vi "HEALTH_LABVIEW_V3.vi"() -> ()   [LabVIEW 2026]
panel:
  out "Waveform Chart":dbl(graph)
  in  "HTR PROP GAIN":dbl=3.0
  in  "PUMP SPEED CONTROL VOLTAGE":dbl(knob) scale=0.0..5.0
  in  "TARGET COOLANT FLOW RATE (LPM)":dbl
  in  "PUMP ON/OFF":bool
  out "HEATER TEMPERATURE (C)":dbl(graph)
  out "HEATER POWER OUTPUT":dbl(knob) scale=0.0..100.0
  in  "TARGET HEATER TEMP (C)":dbl
  in  "HEATER ON/OFF":bool
  out "HEATER TEMP (C)":dbl(knob) scale=20.0..90.0
  out "HEATER TEMP (C)":dbl format="%.2f"
  in  "stop":bool
  out "Error String":string
  out "error out":errorcluster
  out "ConnectionType Out":i32
  out "DeviceType Out":i32
  in  "Identifier":string="LJM_idANY"
  in  "ConnectionType":string="LJM_ctANY"
  in  "DeviceType":string="LJM_dtANY"
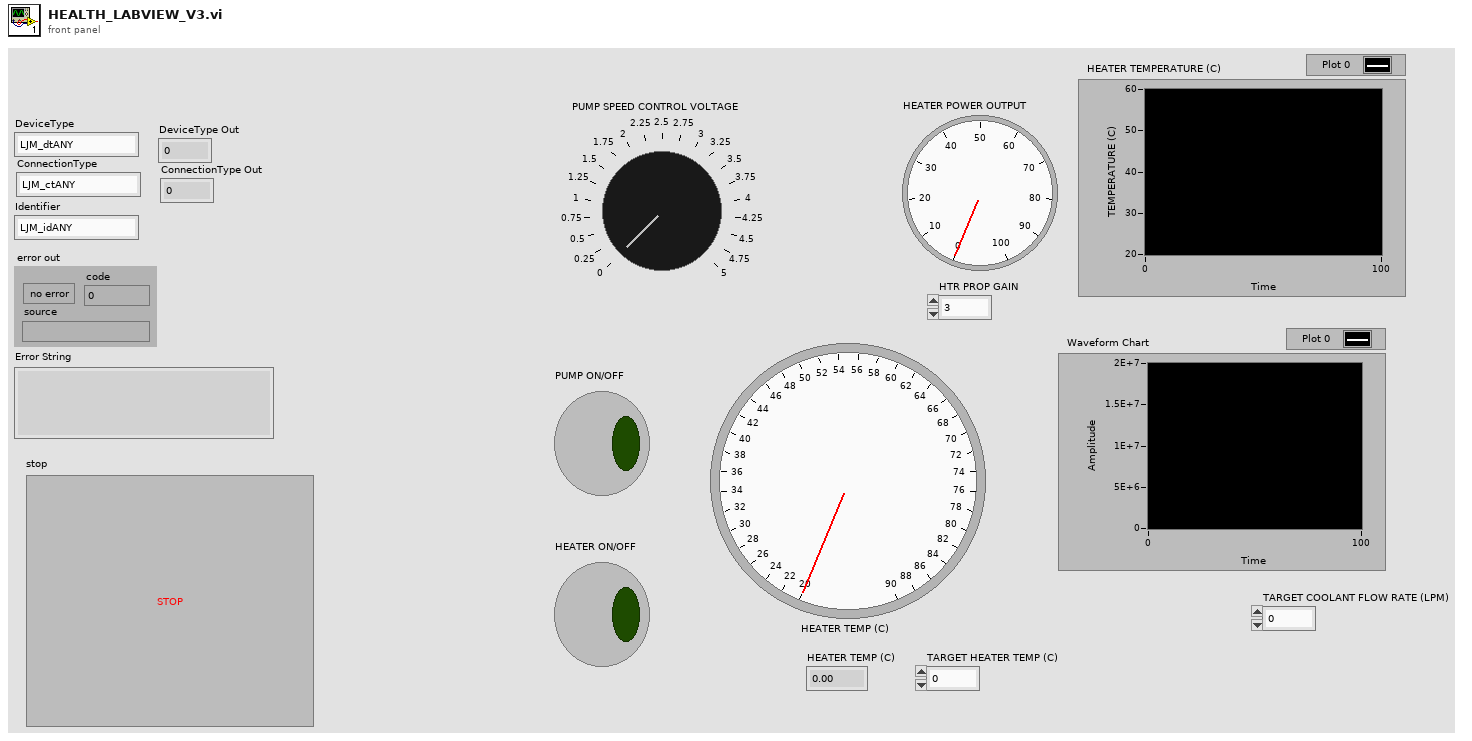
[diagram p1: front panel]
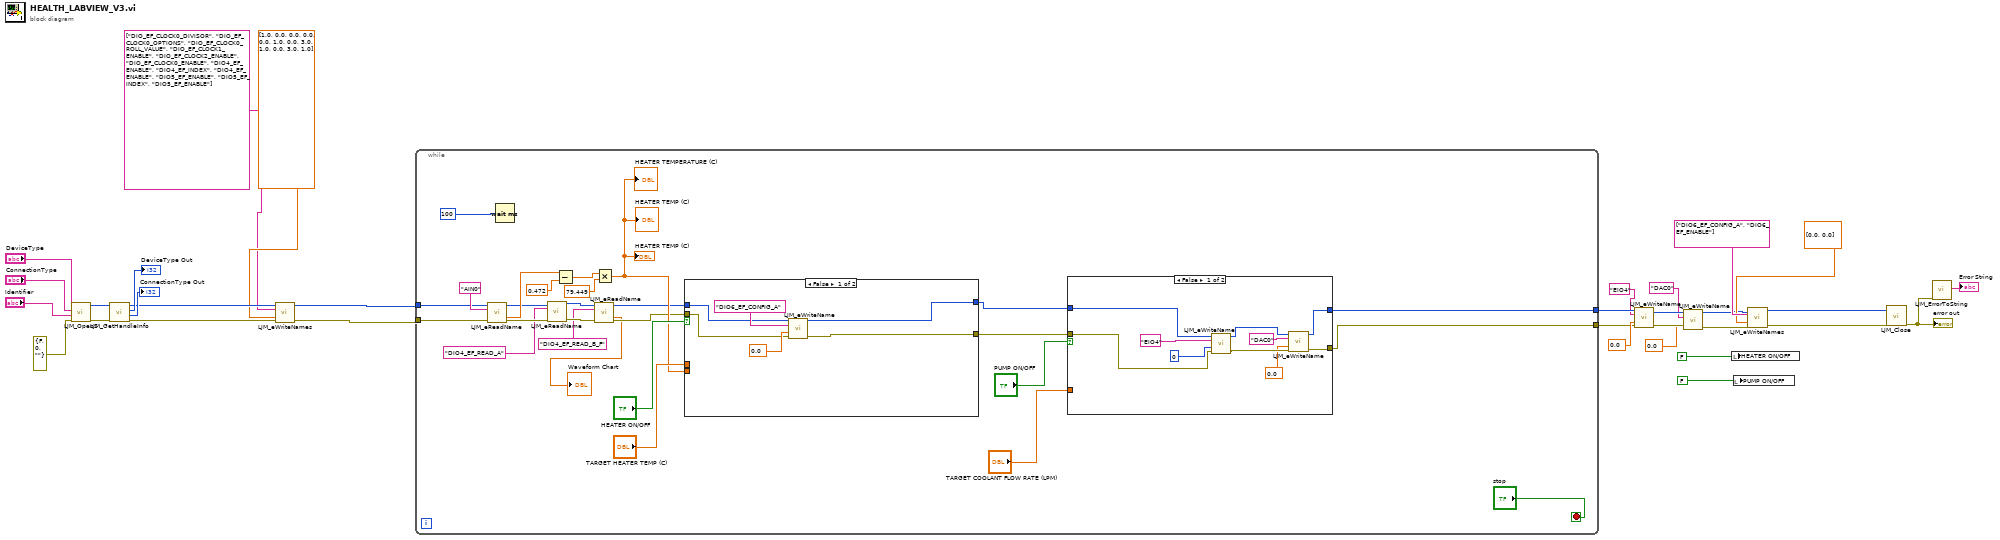
[diagram p0: block diagram]
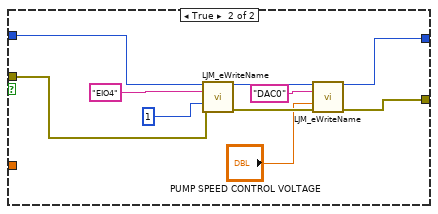
[diagram p2: hidden frame]
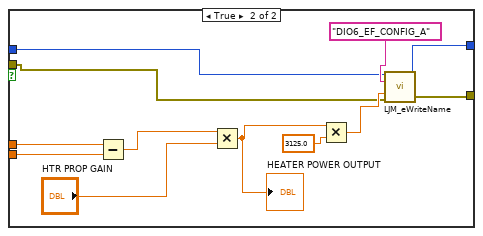
[diagram p3: hidden frame]
diagram:
  n1 = call "LJM_OpenS.vi"("error in"=errorcluster {"status"=FALSE, "code"=0, "source"=""} ("error in (no error)"), "Identifier"="Identifier", "ConnectionType"="ConnectionType", "DeviceType"="DeviceType") -> ("error out"=w31:errorcluster, "Handle"=w30:i32)  [unwired: 6 in]
  n2 = call "LJM_GetHandleInfo.vi"("error in"=w31, "Handle In"=w30) -> ("error out"=w21:errorcluster, "ConnectionType"=→"ConnectionType Out":i32, "DeviceType"=→"DeviceType Out":i32, "Handle Out"=w22:i32)  [unwired: 2 in, 4 out]
  n3 = call "LJM_eWriteNames.vi"("Handle In"=w22, "aNames"=string[] ["DIO_EF_CLOCK0_DIVISOR", "DIO_EF_CLOCK0_OPTIONS", "DIO_EF_CLOCK0_ROLL_VALUE", "DIO_EF_CLOCK1_ENABLE", "DIO_EF_CLOCK2_ENABLE", "DIO_EF_CLOCK0_ENABLE", "DIO4_EF_ENABLE", "DIO4_EF_INDEX", "DIO4_EF_ENABLE", "DIO5_EF_ENABLE", "DIO5_EF_INDEX", "DIO5_EF_ENABLE"], "aValuesIn"=dbl[] [1.0, 0.0, 0.0, 0.0, 0.0, 1.0, 0.0, 3.0, 1.0, 0.0, 3.0, 1.0], "error in"=w21) -> ("Handle Out"=w2:i32, "error out"=w1:errorcluster)  [unwired: 9 in, 1 out]
  n4 = while {
    tunnel: [w45] -> w9
    tunnel: w2 -> [w44]
    tunnel: w1 -> [w43]
    tunnel: [w42] -> w3
    stop <- "stop" stop-if-true
    n5 = call "LJM_eReadName.vi"("Handle In"=w44, "Name"="AIN0", "error in"=w43) -> ("Handle Out"=w41:i32, "Value"=w55:dbl, "error out"=w40:errorcluster)  [unwired: 10 in]
    n6 = Wait (ms)(milliseconds to wait=u32 100) -> ()  [unwired: 1 out]
    n7 = call "LJM_eReadName.vi"("Handle In"=w41, "Name"="DIO4_EF_READ_A", "error in"=w40) -> ("Handle Out"=w39:i32, "error out"=w38:errorcluster)  [unwired: 10 in, 1 out]
    n8 = Subtract(x=w55, y=0.472 ("Address 2")) -> (x-y=w58:dbl)
    n9 = call "LJM_eReadName.vi"("Handle In"=w39, "Name"="DIO4_EF_READ_B_F", "error in"=w38) -> ("Handle Out"=w37:i32, "Value"=→"Waveform Chart":dbl, "error out"=w36:errorcluster)  [unwired: 10 in]
    n10 = Multiply(x=w58, y=79.449 ("Address 2")) -> (x*y=w50:dbl)
    "HEATER TEMP (C)" <- w50
    "HEATER TEMP (C)" <- w50
    "HEATER TEMPERATURE (C)" <- w50
    n11 = case shown="False" "HEATER ON/OFF" {
      tunnel: [w84 w97] -> w46
      tunnel: [w85 w96] -> w47
      tunnel: "TARGET HEATER TEMP (C)" -> [_ w92]
      tunnel: w50 -> [_ w91]
      tunnel: w37 -> [w81 w87]
      tunnel: w36 -> [w80 w86]
      frame False {
        n12 = call "LJM_eWriteName.vi"("Handle In"=w81, "Name"="DIO6_EF_CONFIG_A", "Value"=0.0, "error in"=w80) -> ("Handle Out"=w85:i32, "error out"=w84:errorcluster)  [unwired: 10 in]
      }
      frame True {
        n13 = Subtract(x=w92, y=w91) -> (x-y=w89:dbl)
        n14 = Multiply(x=w89, y="HTR PROP GAIN") -> (x*y=w88:dbl)
        "HEATER POWER OUTPUT" <- w88
        n15 = Multiply(x=w88, y=3125.0) -> (x*y=w94:dbl)
        n16 = call "LJM_eWriteName.vi"("Handle In"=w87, "Name"="DIO6_EF_CONFIG_A", "Value"=w94, "error in"=w86) -> ("Handle Out"=w96:i32, "error out"=w97:errorcluster)  [unwired: 10 in]
      }
    }
    n17 = case shown="False" "PUMP ON/OFF" {
      tunnel: "TARGET COOLANT FLOW RATE (LPM)" -> [_ _]
      tunnel: w47 -> [w67 w77]
      tunnel: w46 -> [w66 w76]
      tunnel: [w62 w71] -> w42
      tunnel: [w61 w72] -> w45
      frame False {
        n18 = call "LJM_eWriteName.vi"("Handle In"=w67, "Name"="EIO4", "Value"=0, "error in"=w66) -> ("Handle Out"=w64:i32, "error out"=w63:errorcluster)  [unwired: 10 in]
        n19 = call "LJM_eWriteName.vi"("Handle In"=w64, "Name"="DAC0", "Value"=0.0, "error in"=w63) -> ("Handle Out"=w61:i32, "error out"=w62:errorcluster)  [unwired: 10 in]
      }
      frame True {
        n20 = call "LJM_eWriteName.vi"("Handle In"=w77, "Name"="EIO4", "Value"=1, "error in"=w76) -> ("Handle Out"=w73:i32, "error out"=w74:errorcluster)  [unwired: 10 in]
        n21 = call "LJM_eWriteName.vi"("Handle In"=w73, "Name"="DAC0", "Value"="PUMP SPEED CONTROL VOLTAGE", "error in"=w74) -> ("Handle Out"=w72:i32, "error out"=w71:errorcluster)  [unwired: 10 in]
      }
    }
  }
  n22 = call "LJM_eWriteName.vi"("Handle In"=w9, "Name"="EIO4", "Value"=0.0, "error in"=w3) -> ("Handle Out"=w10:i32, "error out"=w13:errorcluster)  [unwired: 10 in]
  n23 = call "LJM_eWriteName.vi"("Handle In"=w10, "Name"="DAC0", "Value"=0.0, "error in"=w13) -> ("Handle Out"=w11:i32, "error out"=w12:errorcluster)  [unwired: 10 in]
  n24 = local write "HEATER ON/OFF"(FALSE ("HEATER ON/OFF 2")) -> ()
  n25 = local write "PUMP ON/OFF"(FALSE ("PUMP ON/OFF 2")) -> ()
  n26 = call "LJM_eWriteNames.vi"("Handle In"=w11, "aNames"=string[] ["DIO6_EF_CONFIG_A", "DIO6_EF_ENABLE"], "aValuesIn"=dbl[] [0.0, 0.0], "error in"=w12) -> ("Handle Out"=w17:i32, "error out"=w18:errorcluster)  [unwired: 9 in, 1 out]
  n27 = call "LJM_Close.vi"("error in"=w18, "Handle"=w17) -> ("error out"=w23:errorcluster)  [unwired: 9 in]
  "error out" <- w23
  n28 = call "LJM_ErrorToString.vi"("error in"=w23) -> ("String"=→"Error String":string)  [unwired: 10 in]
